vi "LVClass_CorrectionDataManager ComputeInteractionMatrix.vi"(0 "CorrectionDataManager in":refnum<class "CorrectionDataManager.lvclass">, 7 "HasoSlopes array":refnum<class "HasoSlopes.lvclass">[](array[class]), 11 "error in (no error)":errorcluster) -> (4 "CorrectionDataManager out":refnum<class "CorrectionDataManager.lvclass">, 8 "HasoSlopes array 2":refnum<class "HasoSlopes.lvclass">[](array[class]), 15 "error out":errorcluster)   [LabVIEW 2020, in "CorrectionDataManager.lvclass"]
doc: "Compute interaction matrix from collected calibration data (two HasoSlopes\nmeasured per actuator).\n\n<B>CorrDataManagerIn</B> : CorrDataManager object.\n<B>CorrDataManagerOut</B> : CorrDataManager object.\n<B>HasoSlopes_array_size</B> : Measured HasoSlopes array size (must be 2 x actuators number)\n<B>HasoSlopes_array</B> : HasoSlopes measured for each calibration step."
uses:
  CorrectionDataManager.lvclass
  HasoSlopes.lvclass
  CorrectionDataManager.lvclass/CorrectionDataManager.ctl
  LVClass_HasoSlopes Read HasoSlopes _ property.vi
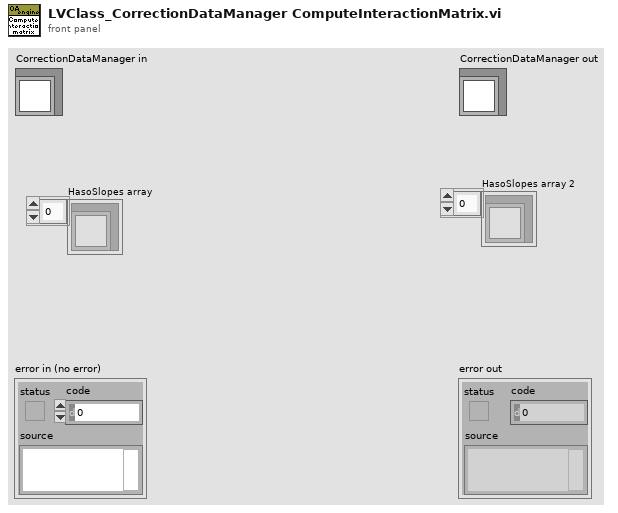
[diagram p1: front panel]
types:
  T1 = typedef "ClassID.ctl" = i64
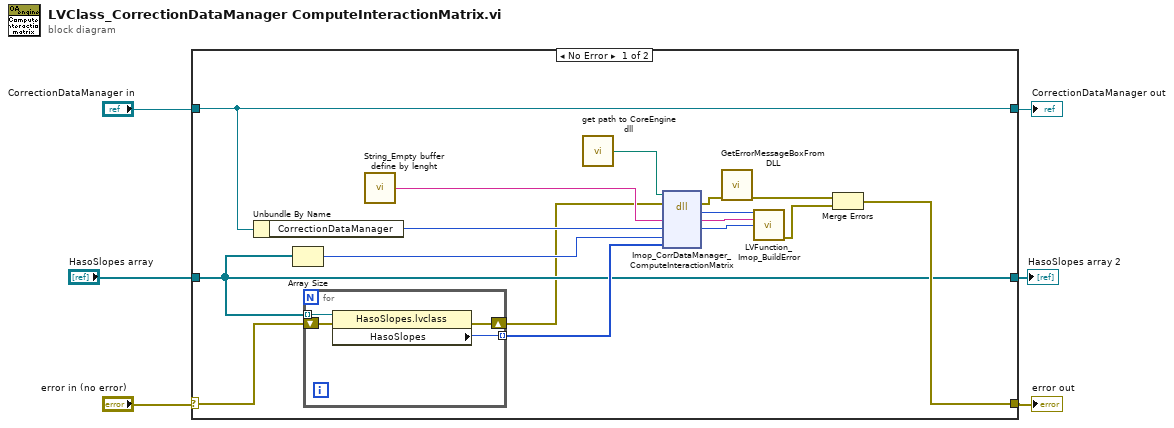
[diagram p0: block diagram]
diagram:
  n1 = case shown="No Error" "error in (no error)" {
    selector: "error in (no error)" -> [w10 w29]
    tunnel: [w15 w29] -> w5
    tunnel: [w13 w28] -> w6
    tunnel: "CorrectionDataManager in" -> [w13 w28]
    tunnel: "HasoSlopes array" -> [w9 w27]
    tunnel: [w9 w27] -> w1
    frame No Error {
      n2 = Unbundle By Name(w13) -> ("CorrectionDataManager"=w14:T1)
      n3 = Array Size(array=w9) -> (size(s)=w11:i32)
      n4 = for {
        tunnel: w9 -> [w25] mode=indexing
        tunnel: [w26] -> w12 mode=indexing
        shift-right: [w23] -> w8
        shift-left: w10 -> [w24]
        n5 = property class="HasoSlopes.lvclass"(reference=w25, error in=w24) -> (error out=w23:errorcluster, "HasoSlopes"=w26:T1)  [unwired: 1 out]
      }
      n6 = call "String_Empty buffer define by lenght.vi"() -> ("Empty buffer"=w20:string)  [unwired: 1 in]
      n7 = call "get path to CoreEngine dll.vi"() -> ("path to wavekit library"=w19:path)  [unwired: 14 in, 1 out]
      n8 = dll-call lib="D:/soft/HASO_v3/SVN_trunk/ImOpCoreEngine4_LV2011/DLLs/c_interface_vc100.dll" fn="Imop_CorrDataManager_ComputeInteractionMatrix"(path in=w19, error in=w8, "message"=w20, "WavefrontCorrection"=w14, "size"=w11, "HasoSlopes array"=w12) -> (error out=w18:errorcluster, "return type"=w22:i32, "message"=w21:string, "WavefrontCorrection"=w7:i64)  [unwired: 3 in, 1 out]
      n9 = call "GetErrorMessageBoxFromDLL.vi"("error IN"=w18) -> ("error OUT"=w17:errorcluster)  [unwired: 10 in]
      n10 = call "LVFunction_Imop_BuildError.vi"("code"=w22, "String to Prepend to source (\"\")"=w21, "Adresse"=w7) -> ("error out"=w16:errorcluster)  [unwired: 12 in]
      n11 = Merge Errors(w17, w16) -> (w15:errorcluster)
    }
    frame Error {
    }
  }
  "error out" <- w5
  "CorrectionDataManager out" <- w6
  "HasoSlopes array 2" <- w1
